vi "GT EQ LT.vi"(1 "基准":dbl, 2 "in":dbl) -> (0 "out":i32)   [LabVIEW 2018]
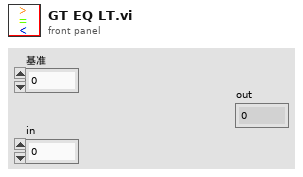
[diagram p1: front panel]
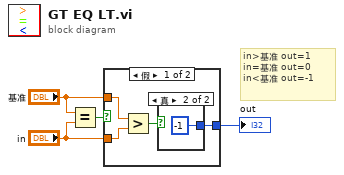
[diagram p0: block diagram]
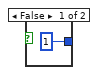
[diagram p2: hidden frame]
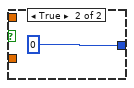
[diagram p3: hidden frame]
diagram:
  # "in>基准 out=1\nin=基准 out=0\nin<基准 out=-1"
  n1 = Equal?(x="基准", y="in") -> (x = y?=w4:bool)
  n2 = case shown="假" w4 {
    tunnel: [w5 0] -> w3
    tunnel: "基准" -> [w8 _]
    tunnel: "in" -> [w7 _]
    frame False {
      n3 = Greater?(x=w8, y=w7) -> (0:w6:bool)
      n4 = case shown="真" w6 {
        tunnel: [1 -1] -> w5
        frame False {
        }
        frame True {
        }
      }
    }
    frame True {
    }
  }
  "out" <- w3
